vi "GenerateRoomReport.vi"(8 "Error In":errorcluster) -> (0 "Error Out":errorcluster, 1 "Update?":bool, 2 "RoomGraphs":T2 {"NurseAvgFulfillTime(s)" scale=0.0..100.0; "DrAvgFulfillTime(s)" scale=0.0..200.0; "#NurseAlarms" scale=0.0..10.0; "#Patients" scale=0.0..10.0; "#DrAlarms" scale=0.0..10.0; "AvgStayPerRoom(s)" scale=0.0..10.0}, 3 "RoomReport":T1)   [LabVIEW 2015]
uses:
  TypeDef/RoomReportGraphs.ctl
  TypeDef/RoomReport.ctl
panel:
  in  "Cancel":bool
  in  "Submit":bool
  in  "Rooms":string[](array[string])
  in  "To":timestamp
  in  "From":timestamp
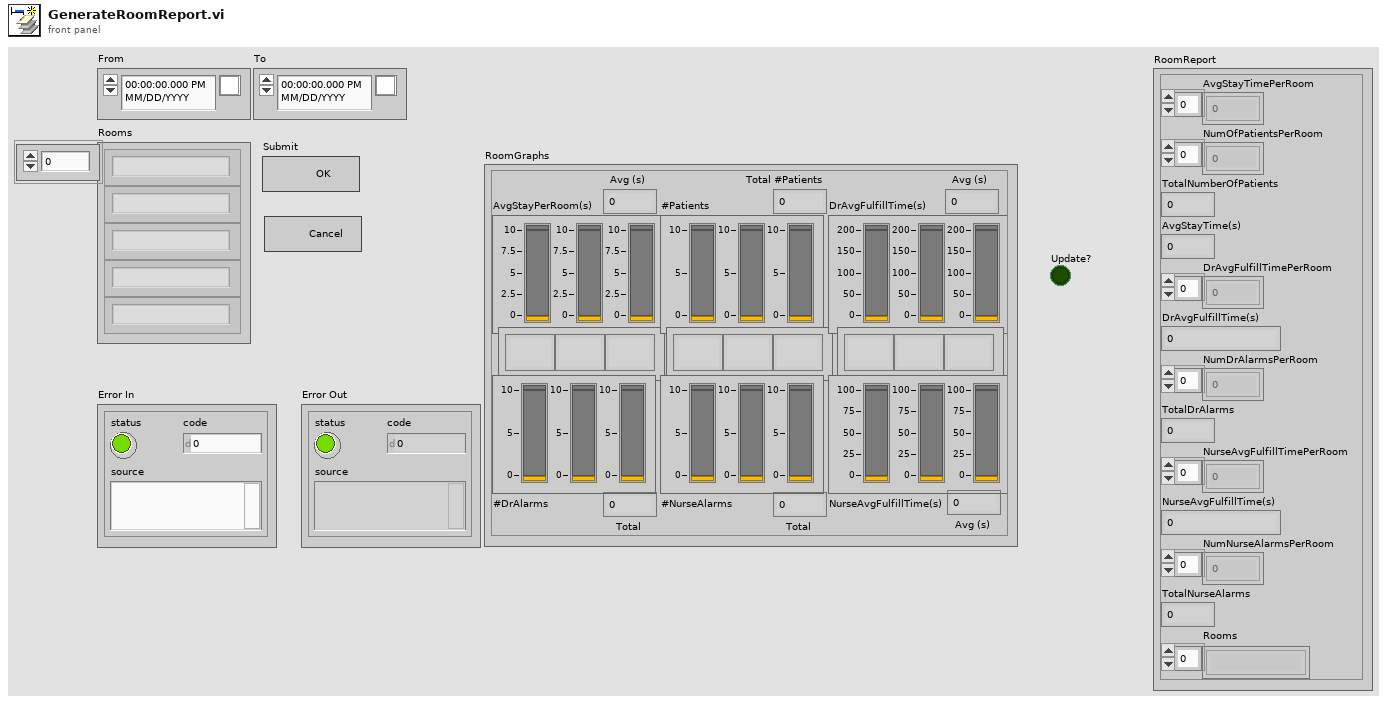
[diagram p1: front panel]
types:
  T1 = typedef "RoomReport.ctl" = cluster{"AvgStayTimePerRoom":dbl[], "NumOfPatientsPerRoom":i32[], "TotalNumberOfPatients":i32, "AvgStayTime(s)":dbl, "DrAvgFulfillTimePerRoom":dbl[], "DrAvgFulfillTime(s)":dbl, "NumDrAlarmsPerRoom":i32[], "TotalDrAlarms":i32, "NurseAvgFulfillTimePerRoom":dbl[], "NurseAvgFulfillTime(s)":dbl, "NumNurseAlarmsPerRoom":i32[], "TotalNurseAlarms":i32, "Rooms":string[]}
  T2 = typedef "RoomReportGraphs.ctl" = cluster{"AvgStay (s)":dbl, "AvgStayPerRoom(s)":dbl[], "Total #Patients":i32, "#Patients":i32[], "TotalDrAvgFulfillTime(s)":dbl, "DrAvgFulfillTime(s)":dbl[], "#DrAlarms":i32[], "TotalDrAlarms":i32, "#NurseAlarms":i32[], "TotalNurseAlarms":i32, "NurseAvgFulfillTime(s)":dbl[], "TotalNurseAvgFulfillTime(s)":dbl, "RoomNumArr1":string[], "RoomNumArr2":string[], "RoomNumArr3":string[]}
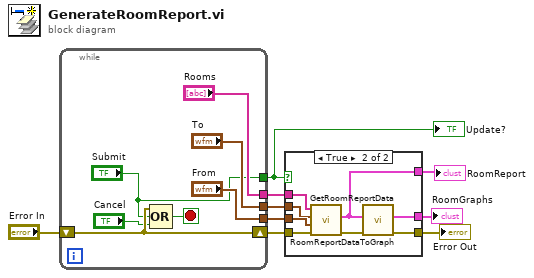
[diagram p0: block diagram]
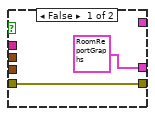
[diagram p2: hidden frame]
diagram:
  n1 = while {
    shift-right: [w12] -> w7
    shift-left: "Error In" -> [w12]
    tunnel: ["From"] -> w5
    tunnel: ["To"] -> w4
    tunnel: ["Rooms"] -> w6
    tunnel: ["Submit"] -> w3
    stop <- w13 stop-if-true
    n2 = Compound Arithmetic op=OR(w12, "Submit", "Cancel") -> (w13:bool)
  }
  "Update?" <- w3
  n3 = case shown="True" w3 {
    tunnel: [w18 w21] -> w8
    tunnel: w7 -> [w18 w25]
    tunnel: w6 -> [_ w24]
    tunnel: w5 -> [_ w23]
    tunnel: w4 -> [_ w22]
    tunnel: [T2 {"AvgStay (s)"=0.0, "AvgStayPerRoom(s)"=[], "Total #Patients"=0, "#Patients"=[], "TotalDrAvgFulfillTime(s)"=0.0, "DrAvgFulfillTime(s)"=[], "#DrAlarms"=[], "TotalDrAlarms"=0, "#NurseAlarms"=[], "TotalNurseAlarms"=0, "NurseAvgFulfillTime(s)"=[], "TotalNurseAvgFulfillTime(s)"=0.0, "RoomNumArr1"=[], "RoomNumArr2"=[], "RoomNumArr3"=[]} ("RoomGraphs") w20] -> w2
    tunnel: [_ w19] -> w1
    frame False {
    }
    frame True {
      n4 = call "GetRoomReportData.vi"("error in"=w25, "From"=w23, "To"=w22, "Rooms"=w24) -> ("error out"=w26:errorcluster, "RoomReport"=w19:T1)  [unwired: 6 in]
      n5 = call "RoomReportDataToGraph.vi"("Error In"=w26, "RoomReport"=w19) -> ("Error Out"=w21:errorcluster, "RoomGraphs"=w20:T2)  [unwired: 8 in]
    }
  }
  "Error Out" <- w8
  "RoomGraphs" <- w2
  "RoomReport" <- w1
